vi "Camera_GUI.vi"(10 "stop 2":refnum<vi>, 11 "GUI_cluster":T1={"Sub Panel"=refnum, "GUIdevice"="Bella_LP_Mode", "CtlRef"=refnum, "User Event in"=refnum}) -> ()   [LabVIEW 2013]
uses:
  Shared/GUI_Template/GUI_master/tcp new data cluster.ctl
  Controls/eventtypdef1.ctl
  Shared/GUI_Template/GUI_master/tcp_new_data_event.ctl
  Controls/GUI_cluster.ctl
panel:
  in  "Target.Y::2":dbl=0.001 caption="targetY" min=0.0 max=2000.0 format="%_1p"
  in  "Target.X::2":dbl=0.001 caption="targetX" min=0.0 max=2000.0 format="%_1p"
  out "tcp data event":T2
  in  "trigger::2":bool caption="Trigger"
  in  "gain::2":dbl=0.001 caption="gain" min=0.0 max=12.0 format="%_1p"
  out "image::2":T3(plugin-control) caption="Mode1"
  in  "exposure::2":dbl=0.001 caption="exposure" min=0.0001 max=1.0 format="%_1p"
  out "GUIdevice 2":string="Bella_LP_Mode"
  in  "stop":bool
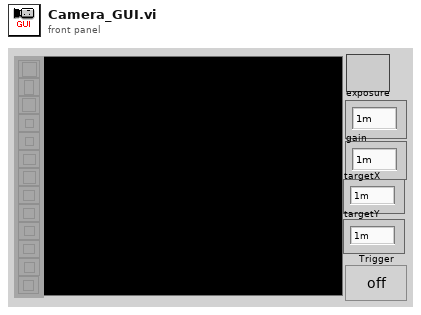
[diagram p1: front panel]
types:
  T1 = typedef "GUI_cluster.ctl" = cluster{"Sub Panel":refnum<vi>, "GUIdevice":string, "CtlRef":refnum<vi>, "User Event in":refnum<user-event>}
  T2 = typedef "tcp_new_data_event.ctl" = refnum<user-event>
  T3 = typedef "IMAQ Image.ctl" = refnum<image>
  T4 = typedef "Image Type" = u32
  T5 = typedef "eventtypdef1.ctl" = cluster{"label":string, "Sub Panel":refnum<vi>, "CtlRef":refnum<vi>, "This VI":refnum<vi>}
  T6 = typedef "tcp new data cluster.ctl" = cluster{"EventEnum":enum16{"new data", "connection status update"}, "Device name":string}
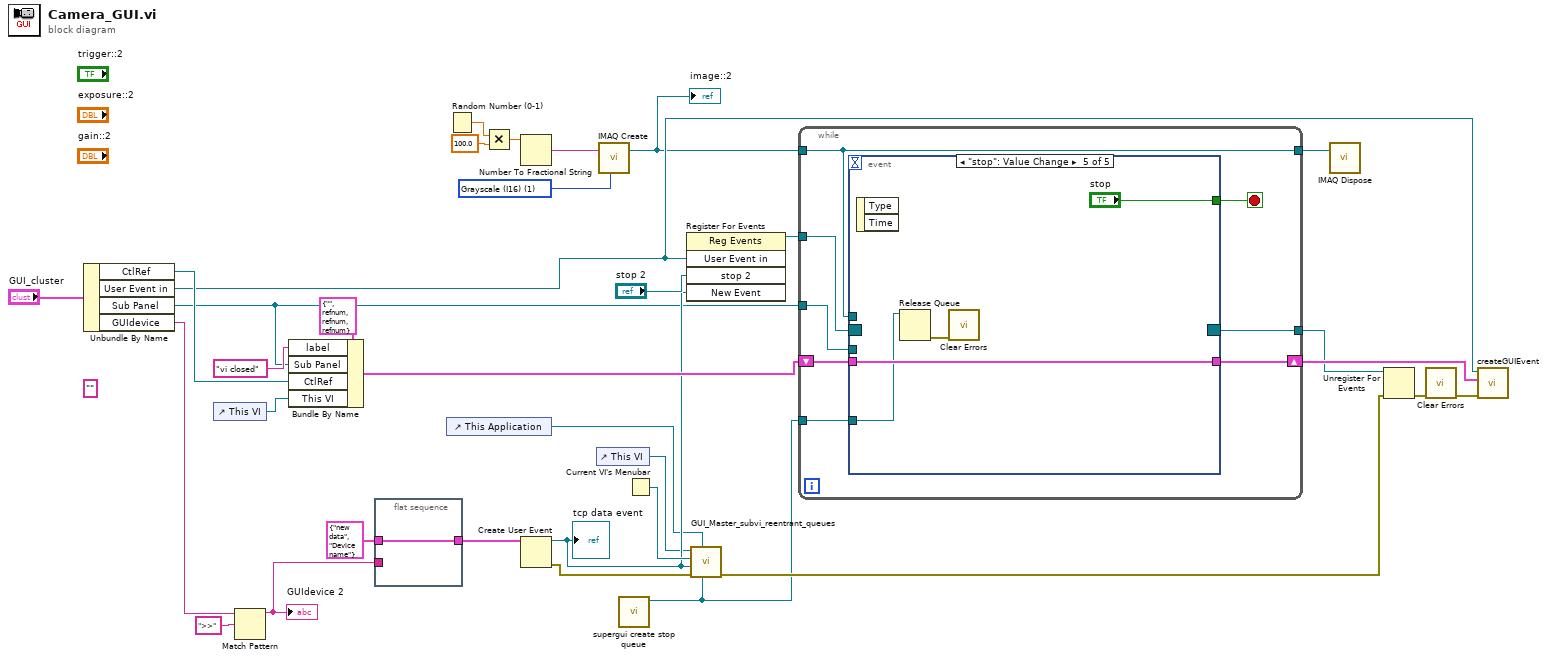
[diagram p0: block diagram]
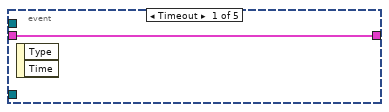
[diagram p2: hidden frame]
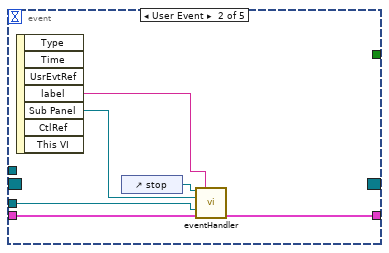
[diagram p3: hidden frame]
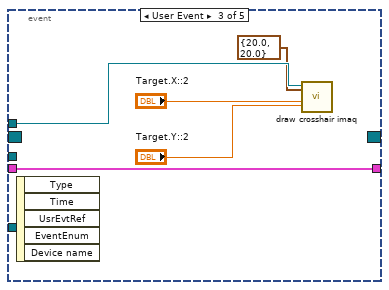
[diagram p4: hidden frame]
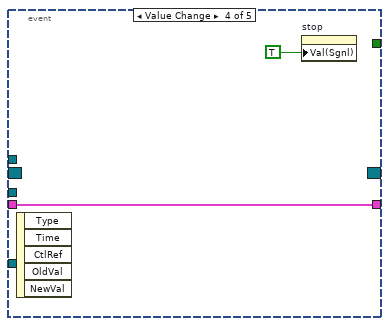
[diagram p5: hidden frame]
diagram:
  w13 = T4 1 items=["Grayscale (U8)", "Grayscale (I16)", "Grayscale (SGL)", "Complex (CSG)", "RGB (U32)", "HSL (U32)", "RGB (U64)", "Grayscale (U16)"] ("Image Type")
  (unwired) ""
  n1 = Unbundle By Name("GUI_cluster") -> ("CtlRef"=w29:refnum<vi>, "User Event in"=w25:refnum<user-event>, "Sub Panel"=w5:refnum<vi>, "GUIdevice"=w28:string)
  n2 = control-ref of="This VI"() -> (w4:refnum<vi>)
  n3 = Match Pattern(string=w28, regular expression=">>") -> (before substring=w2:string)  [unwired: 1 in, 3 out]
  "GUIdevice 2" <- w2
  n4 = Bundle By Name(cluster=T5 {"label"="", "Sub Panel"=refnum, "CtlRef"=refnum, "This VI"=refnum} ("event data"), "label"="vi closed", "Sub Panel"=w5, "CtlRef"=w29, "This VI"=w4) -> (w23:T5)
  n5 = flat-sequence {
    tunnel: T6 {"EventEnum"=enum."new data", "Device name"="Device name"} ("New Event") -> [w34]
    tunnel: [w34] -> w20
    tunnel: w2 -> [_]
    frame #0 {
    }
  }
  n6 = Random Number (0-1)() -> (number: 0 to 1=w17:dbl)
  n7 = control-ref of="This Application"() -> (w11:refnum<vi>)
  n8 = Multiply(x=w17, y=100.0) -> (x*y=w15:dbl)
  n9 = Number To Fractional String(number=w15) -> (F-format string=w3:string)  [unwired: 3 in]
  n10 = Create User Event(user event datatype=w20) -> (user event=w18:refnum<user-event>, error out=w32:errorcluster)  [unwired: 1 in]
  "tcp data event" <- w18
  n11 = control-ref of="This VI"() -> (w10:refnum<vi>)
  n12 = call "IMAQ Create"("Image Name"=w3, "Image Type"=w13) -> ("New Image"=w14:T3)  [unwired: 3 in, 1 out]
  "image::2" <- w14
  n13 = call "supergui create stop queue.vi"() -> ("STOP Queue out"=w1:refnum<queue>)  [unwired: 11 in]
  n14 = Current VI's Menubar() -> (w33:refnum<k9>)
  n15 = register-events(w25, "stop 2", w18) -> (reference out=w26:refnum<event-registration>)  [unwired: 2 in, 1 out]
  n16 = call "GUI_Master_subvi_reentrant_queues.vi"("STOP Queue in"=w1, "This Application"=w11, "error in (no error)"=w32, "tcp data event"=w18, "Caller menu reference"=w33, "Caller VI ref"=w10) -> ("error out"=w7:errorcluster)  [unwired: 5 in]
  n17 = while {
    tunnel: w26 -> [w42]
    tunnel: w5 -> [w40]
    shift-right: [w38] -> w22
    shift-left: w23 -> [w39]
    tunnel: w14 -> [w37]
    tunnel: [w37] -> w12
    tunnel: [w36] -> w8
    tunnel: w1 -> [w35]
    stop <- w41 stop-if-true
    n18 = event shown="[4] \"stop\": Value Change" {
      selector: w42 -> [_ _ _ _ _]
      dyn-events: [_ _ _ _ _] -> w36
      timeout: _ -> [_ _ _ _ _]
      tunnel: [_ _ _ _ "stop"] -> w41
      tunnel: w40 -> [_ w46 _ _ _]
      tunnel: w39 -> [w43 w45 w54 w55 w59]
      tunnel: [w43 w44 w54 w55 w59] -> w38
      tunnel: w37 -> [_ _ w53 _ _]
      tunnel: w35 -> [_ _ _ _ w57]
      event Timeout {
        n19 = event-data() -> ()  [unwired: 1 in, 2 out]
      }
      event User Event {
        n20 = event-data() -> ("label"=w49:string, "Sub Panel"=w48:refnum<vi>)  [unwired: 1 in, 5 out]
        n21 = control-ref of="stop"() -> (w47:refnum<vi>)
        n22 = call "eventHandler.vi"("Boolean in"=w47, "label"=w49, "Sub Panel 2"=w48, "Sub Panel"=w46, "event data in"=w45) -> ("event data out"=w44:T5)  [unwired: 10 in]
      }
      event User Event {
        n23 = event-data() -> ()  [unwired: 1 in, 5 out]
        n24 = call "draw crosshair imaq.vi"(6:"Target.Y::2", "clear overlay"=cluster{"xhair size":dbl, "xhair size 2":dbl} {"xhair size"=20.0, "xhair size 2"=20.0} ("size"), "Crosshair"="Target.X::2", "image in"=w53) -> ()  [unwired: 6 in, 2 out]
      }
      event Value Change {
        n25 = event-data() -> ()  [unwired: 1 in, 5 out]
        n26 = property on="stop" class="Bool (strict)"("Val(Sgnl)"=TRUE ("Value (Signaling)")) -> ()  [unwired: 2 in, 2 out]
      }
      event "stop": Value Change {
        n27 = event-data() -> ()  [unwired: 1 in, 2 out]
        n28 = Release Queue(queue=w57) -> (error out=w58:errorcluster)  [unwired: 2 in, 2 out]
        n29 = call <vilib>:"Clear Errors.vi"("error in (no error)"=w58) -> ()  [unwired: 6 in, 1 out]
      }
    }
  }
  n30 = call "IMAQ Dispose"("Image"=w12) -> ()  [unwired: 5 in, 1 out]
  n31 = Unregister For Events(event registration refnum=w8, error in=w7) -> (error out=w9:errorcluster)
  n32 = call <vilib>:"Clear Errors.vi"("error in (no error)"=w9) -> ("error out"=w6:errorcluster)  [unwired: 6 in]
  n33 = call "createGUIEvent.vi"("error in (no error)"=w6, "event data"=w22, "User Event in"=w25) -> ()  [unwired: 8 in, 1 out]
